vi "WILT Find Start Button.vi"(10 "Agilent Valve and Switch Locations":T1[](array[typedef]), 11 "Station Number":i32) -> (1 "Channel":string, 2 "Agilent Station":string, 3 "Station Number":i32, 4 "Label":string)   [LabVIEW 2016]
uses:
  Type Definitions/WILT Agilent Channel Definition.ctl
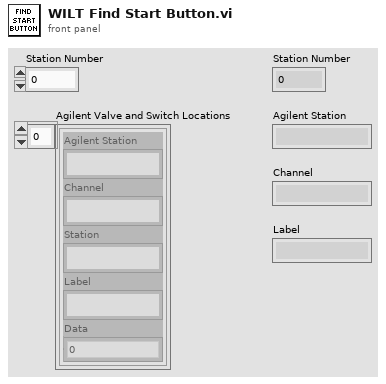
[diagram p1: front panel]
types:
  T1 = typedef "WILT Agilent Channel Definition.ctl" = cluster{"Channel":string, "Station":string, "Label":string, "Agilent Station":string, "Data":dbl}
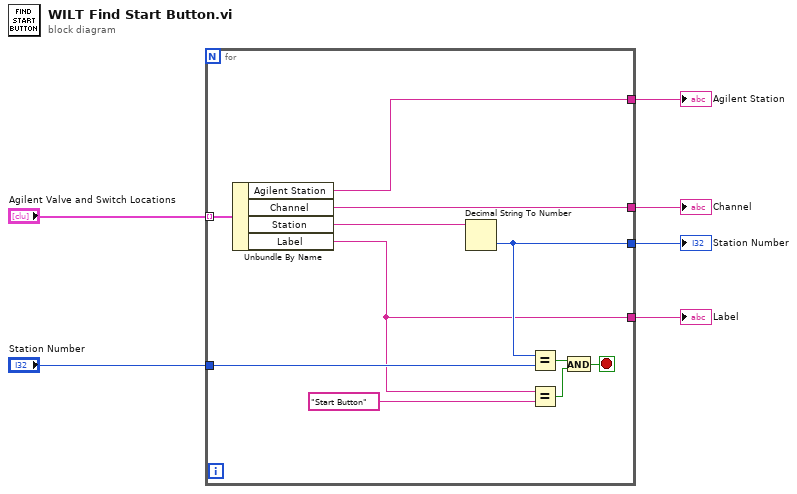
[diagram p0: block diagram]
diagram:
  n1 = for {
    tunnel: "Agilent Valve and Switch Locations" -> [w17] mode=indexing
    tunnel: [w16] -> w3
    tunnel: [w15] -> w4
    tunnel: "Station Number" -> [w12]
    tunnel: [w8] -> w5
    tunnel: [w7] -> w6
    stop <- w9 stop-if-true
    n2 = Unbundle By Name(w17) -> ("Agilent Station"=w16:string, "Channel"=w15:string, "Station"=w14:string, "Label"=w7:string)
    n3 = Decimal String To Number(string=w14) -> (number=w8:i32)  [unwired: 2 in, 1 out]
    n4 = Equal?(x=w8, y=w12) -> (x = y?=w10:bool)
    n5 = Equal?(x=w7, y="Start Button") -> (x = y?=w11:bool)
    n6 = And(x=w10, y=w11) -> (x .and. y?=w9:bool)
  }
  "Label" <- w6
  "Station Number" <- w5
  "Channel" <- w4
  "Agilent Station" <- w3
